vi "Switch Compare.vi"(8 "Error In":errorcluster, 10 "Switch Position":string, 11 "Alliance Position":dbl) -> (0 "Error Out":errorcluster, 3 "Switch Compare?":bool)   [LabVIEW 2017]
panel:
  # "SWITCH COMPARE"
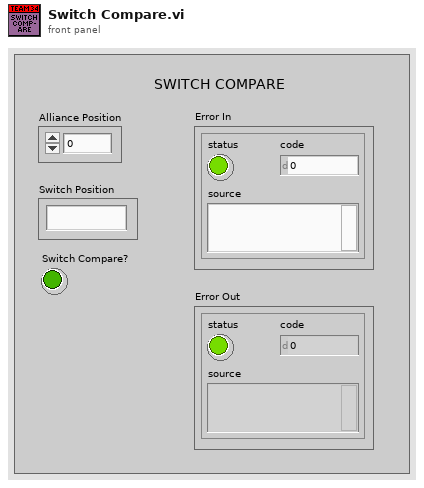
[diagram p1: front panel]
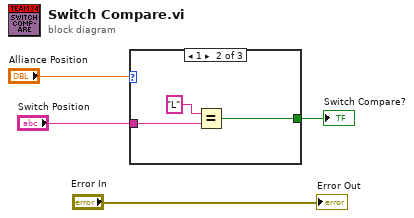
[diagram p0: block diagram]
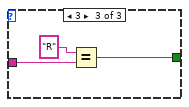
[diagram p3: hidden frame]
diagram:
  n1 = case shown="1" "Alliance Position" {
    tunnel: "Switch Position" -> [_ w6 w10]
    tunnel: [_ w7 w9] -> w4
    frame Default {
    }
    frame 1 {
      n2 = Equal?(x="L", y=w6) -> (x = y?=w7:bool)
    }
    frame 3 {
      n3 = Equal?(x="R", y=w10) -> (x = y?=w9:bool)
    }
  }
  "Switch Compare?" <- w4
  "Error Out" <- "Error In"
